vi "generate filenames to save.vi"(8 "filename (adds .mat)":string="mydata", 11 "path":path=path "C:/Users/QDM2exp/Documents/PK/practiceData") -> (0 "header path":path, 3 "matlab path":path)   [LabVIEW 2019]
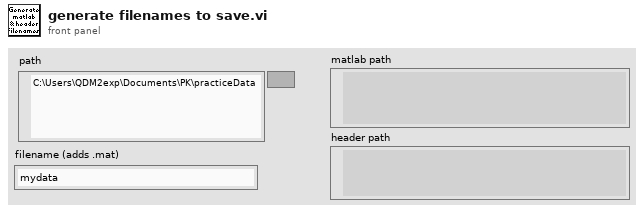
[diagram p1: front panel]
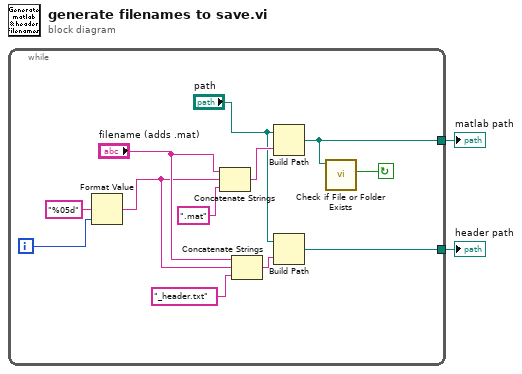
[diagram p0: block diagram]
diagram:
  n1 = while {
    tunnel: [w4] -> w1
    tunnel: [w3] -> w2
    i -> [w14]
    stop <- w11 continue-if-true
    n2 = Format Value(format string="%05d", value (0)=w14) -> (output string=w6:string)  [unwired: 1 in]
    n3 = Concatenate Strings("filename (adds .mat)", w6, ".mat" ("string")) -> (w10:string)
    n4 = Concatenate Strings("filename (adds .mat)", w6, "_header.txt" ("string")) -> (w9:string)
    n5 = Build Path(base path="path", name or relative path=w10) -> (appended path=w3:path)
    n6 = Build Path(base path="path", name or relative path=w9) -> (appended path=w4:path)
    n7 = call <vilib>:"Check if File or Folder Exists.vi"("path"=w3) -> ("file or folder exists?"=w11:bool)  [unwired: 8 in, 2 out]
  }
  "matlab path" <- w2
  "header path" <- w1
